vi "Trapezoidal Acceleration.vi"(6 "Skip":dbl, 8 "AccelRate":dbl, 9 "Desired":dbl, 10 "Actual":dbl, 11 "LoopTime":dbl) -> (2 "New Actual":dbl)   [LabVIEW 2013]
doc: "Fixes motor acceleration to a linear rate."
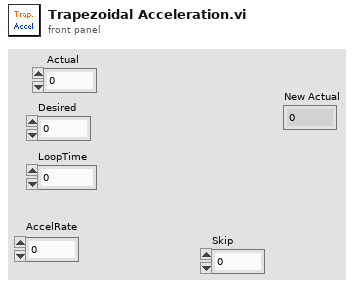
[diagram p1: front panel]
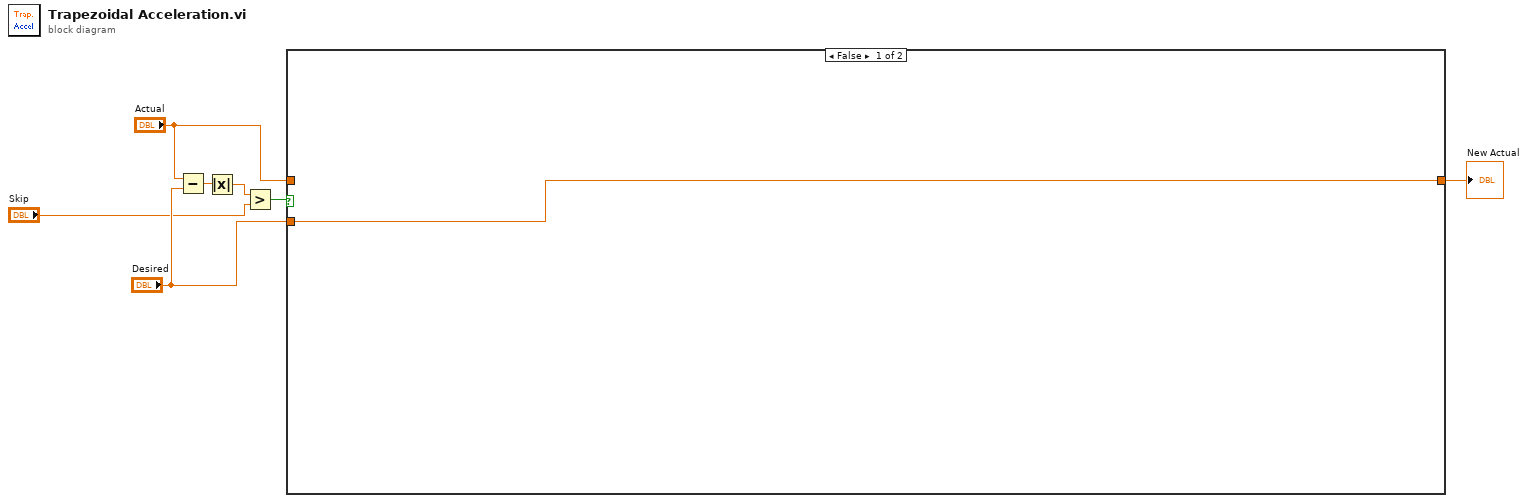
[diagram p0: block diagram]
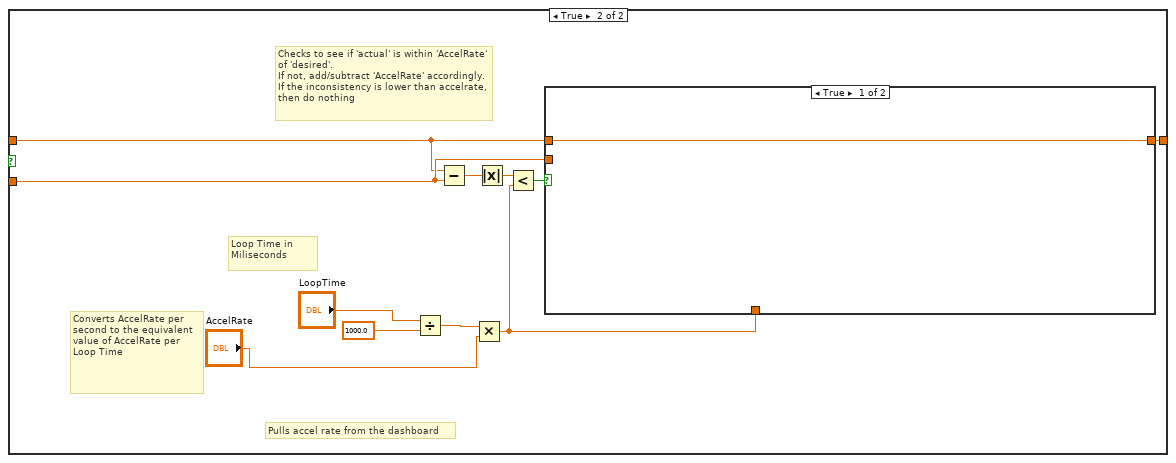
[diagram p2: hidden frame]
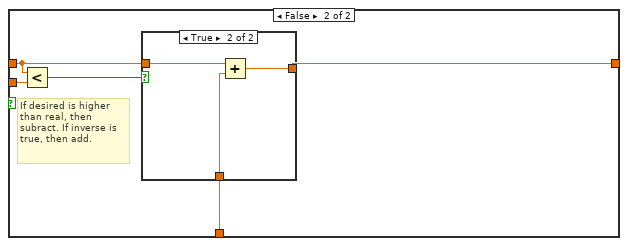
[diagram p3: hidden frame]
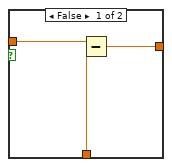
[diagram p4: hidden frame]
diagram:
  n1 = Subtract(x="Actual", y="Desired") -> (x-y=w4:dbl)
  n2 = Absolute Value(x=w4) -> (abs(x)=w2:dbl)
  n3 = Greater?(x=w2, y="Skip") -> (0:w3:bool)
  n4 = case shown="False" w3 {
    tunnel: [w8 w13] -> w7
    tunnel: "Desired" -> [w8 w12]
    tunnel: "Actual" -> [_ w11]
    frame False {
    }
    frame True {
      # "Pulls accel rate from the dashboard"
      # "Checks to see if 'actual' is within 'AccelRate' of 'desired'.\nIf not, add/subtract 'AccelRate' accordingly. If the inconsistency is lower than accelrate, then do nothing"
      # "Converts AccelRate per second to the equivalent value of AccelRate per Loop Time"
      # "Loop Time in Miliseconds"
      n5 = Divide(x="LoopTime", y=1000.0) -> (x/y=w15:dbl)
      n6 = Subtract(x=w11, y=w12) -> (x-y=w18:dbl)
      n7 = Multiply(x=w15, y="AccelRate") -> (x*y=w14:dbl)
      n8 = Absolute Value(x=w18) -> (abs(x)=w19:dbl)
      n9 = Less?(x=w19, y=w14) -> (x < y?=w17:bool)
      n10 = case shown="True" w17 {
        tunnel: [w20 w25] -> w13
        tunnel: w11 -> [w20 w24]
        tunnel: w12 -> [_ w22]
        tunnel: w14 -> [_ w21]
        frame True {
        }
        frame False {
          # "If desired is higher than real, then subract. If inverse is true, then add."
          n11 = Less?(x=w24, y=w22) -> (x < y?=w23:bool)
          n12 = case shown="True" w23 {
            tunnel: w24 -> [w26 w30]
            tunnel: [w28 w31] -> w25
            tunnel: w21 -> [w27 w29]
            frame False {
              n13 = Subtract(x=w26, y=w27) -> (x-y=w28:dbl)
            }
            frame True {
              n14 = Add(x=w30, y=w29) -> (x+y=w31:dbl)
            }
          }
        }
      }
    }
  }
  "New Actual" <- w7
